vi "Initialize Andor Camera.vi"(8 "error in (no error)":errorcluster) -> (0 "Error Out 2":errorcluster, 1 "Drv Success?":i32)   [LabVIEW 2014]
uses:
  Globals/Initilize Globals.vi
  Library Files - Andor and MadCity/Andorlib/atmcd32d.lvlib
panel:
  out "Fastest VS Speed":sgl
  out "VS Speed":sgl[](array[numeric])
  out "pre-amp gains":sgl[](array[numeric])
  out "#preamp gains":i32
  out "# amplifiers":i32
  out "HS Speeds per channel":sgl[][](array[numeric])
  out "Bit Depth per channel":i32[](array[numeric])
  out "#ADC Channels":i32
  out "Lowest EM gain":i32
  out "Highest EM gain":i32
  out "Head Model":string
  out "eprom out":u32
  out "Camera Serial #":i32
  out "PCB version #":u32
  out "Directory Out":string
  out "Camera FirmWare Version":i32
  out "Y-pixels":u32
  out "X-pixels":u32
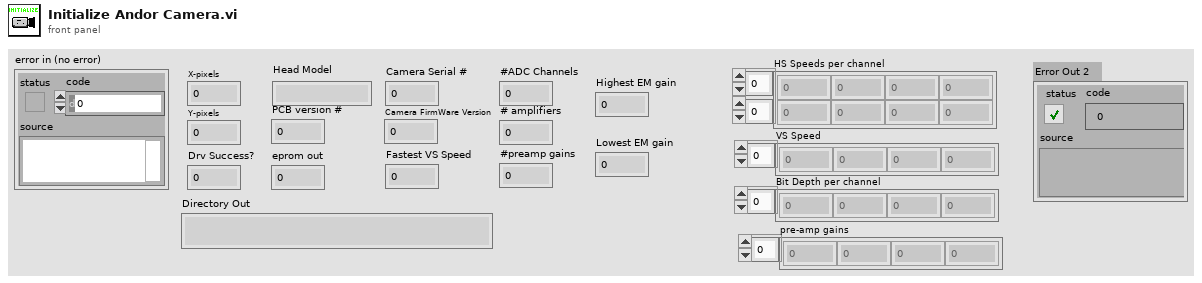
[diagram p1: front panel]
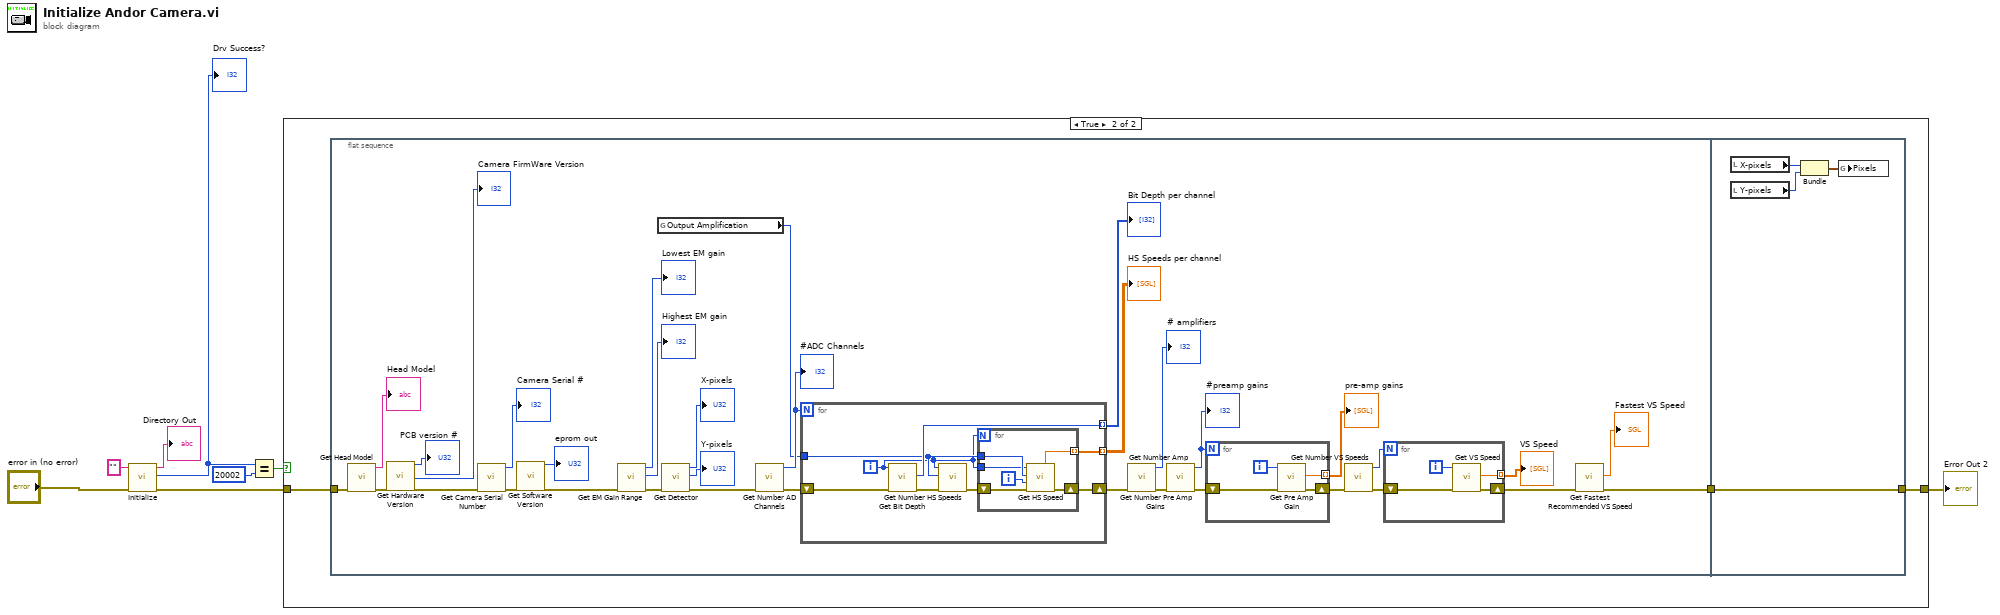
[diagram p0: block diagram]
diagram:
  n1 = call "Initialize.vi"("error in (no error)"="error in (no error)", "dir"="") -> ("error out"=w7:errorcluster, "function return"=w3:u32, "dir out"=→"Directory Out":string)  [unwired: 7 in]
  "Drv Success?" <- w3
  n2 = Equal?(x=w3, y=20002) -> (x = y?=w4:bool)
  n3 = case shown="True" w4 {
    tunnel: [w9 w10] -> w8
    tunnel: w7 -> [w9 w12]
    frame False {
    }
    frame True {
      n4 = flat-sequence {
        tunnel: w12 -> [w38]
        tunnel: [w13] -> w11
        tunnel: [w69] -> w10
        tunnel: w11 -> [w69]
        frame #0 {
          n5 = call "Get Head Model.vi"("error in (no error)"=w38) -> ("error out"=w36:errorcluster, "name out"=→"Head Model":string)  [unwired: 8 in, 1 out]
          n6 = call "Get Hardware Version.vi"("error in (no error)"=w36) -> ("PCB out"=→"PCB version #":u32, "CameraFirmwareVersion out"=→"Camera FirmWare Version":u32, "error out"=w42:errorcluster)  [unwired: 19 in, 5 out]
          n7 = call "Get Camera Serial Number.vi"("error in (no error)"=w42) -> ("error out"=w40:errorcluster, "number out"=→"Camera Serial #":i32)  [unwired: 8 in, 1 out]
          n8 = call "Get Software Version.vi"("error in (no error)"=w40) -> ("eprom out"=→"eprom out":u32, "error out"=w34:errorcluster)  [unwired: 19 in, 6 out]
          n9 = call "Get EM Gain Range.vi"("error in (no error)"=w34) -> ("error out"=w33:errorcluster, "high out"=→"Highest EM gain":i32, "low out"=→"Lowest EM gain":i32)  [unwired: 7 in, 1 out]
          n10 = global read "Initilize Globals.vi" "Output Amplification"() -> (w27:i32)
          n11 = call "Get Detector.vi"("error in (no error)"=w33) -> ("error out"=w35:errorcluster, "ypixels out"=→"Y-pixels":i32, "xpixels out"=→"X-pixels":i32)  [unwired: 7 in, 1 out]
          n12 = call "Get Number AD Channels.vi"("error in (no error)"=w35) -> ("error out"=w29:errorcluster, "channels out"=w30:i32)  [unwired: 8 in, 1 out]
          "#ADC Channels" <- w30
          n13 = for {
            N: w30 -> [_]
            shift-right: [w58] -> w25
            shift-left: w29 -> [w62]
            tunnel: [w61] -> w28 mode=indexing
            tunnel: w27 -> [w56]
            tunnel: [w57] -> w26 mode=indexing
            i -> [w55]
            n14 = call "Get Bit Depth.vi"("error in (no error)"=w62, "channel"=w55) -> ("error out"=w60:errorcluster, "depth out"=w61:i32)  [unwired: 7 in, 1 out]
            n15 = call "Get Number HS Speeds.vi"("error in (no error)"=w60, "typ"=w56, "channel"=w55) -> ("error out"=w59:errorcluster)  [unwired: 6 in, 2 out]
            n16 = for {
              N: w55 -> [_]
              shift-right: [w66] -> w58
              shift-left: w59 -> [w67]
              tunnel: [w65] -> w57 mode=indexing
              tunnel: w56 -> [w64]
              tunnel: w55 -> [w63]
              i -> [w68]
              n17 = call "Get HS Speed.vi"("error in (no error)"=w67, "index"=w68, "typ"=w64, "channel"=w63) -> ("error out"=w66:errorcluster, "speed out"=w65:sgl)  [unwired: 5 in, 1 out]
            }
          }
          "Bit Depth per channel" <- w28
          "HS Speeds per channel" <- w26
          n18 = call "Get Number Amp.vi"("error in (no error)"=w25) -> ("error out"=w23:errorcluster, "amp out"=→"# amplifiers":i32)  [unwired: 8 in, 1 out]
          n19 = call "Get Number Pre Amp Gains.vi"("error in (no error)"=w23) -> ("error out"=w22:errorcluster, "noGains out"=w21:i32)  [unwired: 8 in, 1 out]
          "#preamp gains" <- w21
          n20 = for {
            N: w21 -> [_]
            shift-right: [w53] -> w19
            shift-left: w22 -> [w54]
            tunnel: [w51] -> w20 mode=indexing
            i -> [w52]
            n21 = call "Get Pre Amp Gain.vi"("error in (no error)"=w54, "index"=w52) -> ("error out"=w53:errorcluster, "gain out"=w51:sgl)  [unwired: 7 in, 1 out]
          }
          "pre-amp gains" <- w20
          n22 = call "Get Number VS Speeds.vi"("error in (no error)"=w19) -> ("error out"=w18:errorcluster, "speeds out"=w17:i32)  [unwired: 8 in, 1 out]
          n23 = for {
            N: w17 -> [_]
            shift-right: [w49] -> w15
            shift-left: w18 -> [w50]
            tunnel: [w47] -> w16 mode=indexing
            i -> [w48]
            n24 = call "Get VS Speed.vi"("error in (no error)"=w50, "index"=w48) -> ("error out"=w49:errorcluster, "speed out"=w47:sgl)  [unwired: 7 in, 1 out]
          }
          "VS Speed" <- w16
          n25 = call "Get Fastest Recommended VS Speed.vi"("error in (no error)"=w15) -> ("error out"=w13:errorcluster, "speed out"=→"Fastest VS Speed":sgl)  [unwired: 7 in, 2 out]
        }
        frame #1 {
          n26 = local read "X-pixels"() -> (w71:u32)
          n27 = local read "Y-pixels"() -> (w70:u32)
          n28 = Bundle("X-pixels"=w71, "Y-pixels"=w70) -> (w72:cluster{"X-pixels":u32, "Y-pixels":u32})  [unwired: 1 in]
          n29 = global write "Initilize Globals.vi" "Pixels"(w72) -> ()
        }
      }
    }
  }
  "Error Out 2" <- w8
